vi "TC01_Temp.vi"() -> ()   [LabVIEW 2022 SP3]
panel:
  out "Waveform Chart":dynamicdata(graph)
  out "data":dbl
  out "error out":errorcluster
  in  "stop (F)":bool
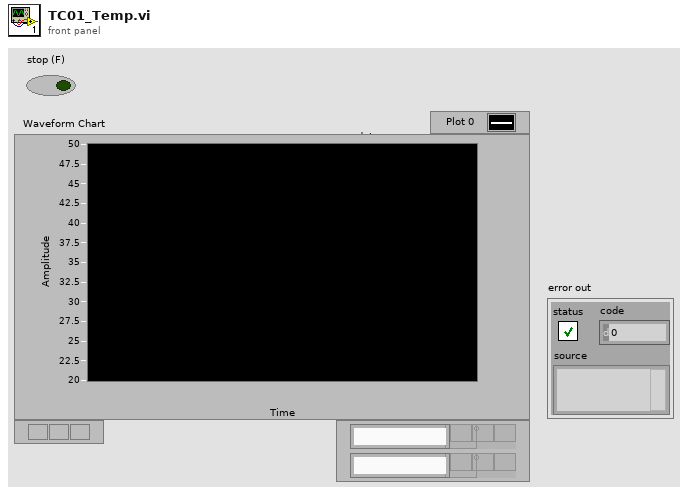
[diagram p1: front panel]
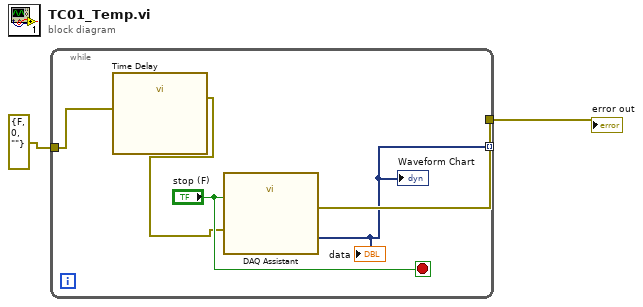
[diagram p0: block diagram]
diagram:
  n1 = while {
    tunnel: [w5] -> _ mode=indexing
    tunnel: errorcluster {"status"=FALSE, "code"=0, "source"=""} ("error in") -> [w4]
    tunnel: [w7] -> w1
    stop <- "stop (F)" stop-if-true
    n2 = call "Time Delay"("error in (no error)"=w4) -> ("error out"=w3:errorcluster)  [unwired: 10 in]
    n3 = call "DAQ Assistant"("error in"=w3, "stop (F)"="stop (F)") -> ("data"=w5:dynamicdata, "error out"=w7:errorcluster)  [unwired: 15 in, 1 out]
    "data" <- w5
    "Waveform Chart" <- w5
  }
  "error out" <- w1
